vi "EnergyMeter Read.vi"(3 "错误输入（无错误）":errorcluster) -> (0 "通信正常？":bool, 1 "错误输出":errorcluster, 2 "能量计读数":string)   [LabVIEW 2018]
uses:
  InOut/Reslut.vi
panel:
  out "Unit":string
  out "能量计输出":dbl
  out "结果字符串":string
  out "数据输出":string
  # "通道A为功率计"
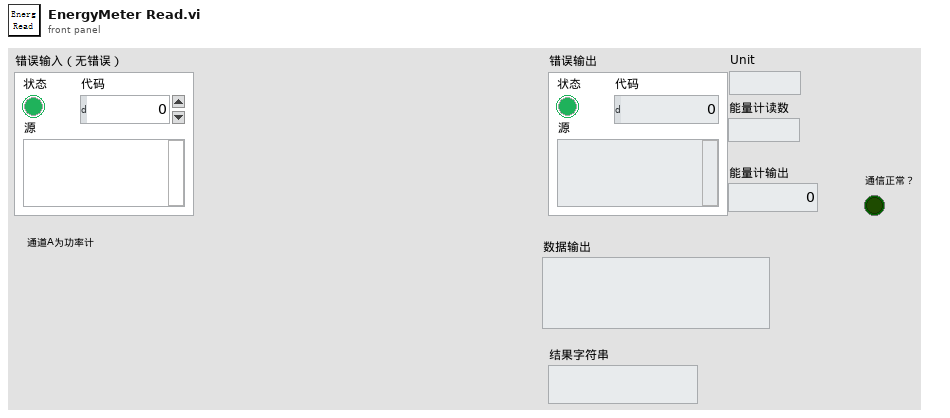
[diagram p1: front panel]
types:
  T1 = enum16{"Standard", "Buffered", "CRLF", "Immediate"}
  T2 = typedef "IMAQ Image.ctl" = refnum<image>
  T3 = cluster{"示波器":cluster{"Channel (0:Channel 1)":enum16{"Channel 1", "Channel 2", "Channel 3", "Channel 4"}, "电压范围":dbl, "触发电压":dbl, "时间范围":dbl, " 示波器VISA":refnum<visa-resource-name>}, "光谱仪":cluster{"Channel (0:Channel 1)":enum16{"Channel 1", "Channel 2", "Channel 3", "Channel 4"}, "电压范围":u64, "触发电压":u64, "时间范围":u64}, " 近场相机":cluster{"曝光时间":i32, "模拟增益":i32, "控制套接字":i32, "IP 地址":string, " 采集套接字":i32, "  版本号":i32, "ImageData":T2, "  增益最大":i32, "  增益最小":i32, " 曝光最大":i32, " 曝光最小":i32, " 帧速":i32, " 同步切换":i32, "  曝光缩放":i32}, " 偏振仪":cluster{"电压范围":u64, "触发电压":u64, "时间范围":u64, "波长范围":enum16{"可见光 400-700nm", "近红外 700-1100nm"}}, " 功率计":cluster{"通道":enum16{"Channel 1", "Channel 2"}, "工作波长":u32, "单位":u64, "时间范围":u64, "IP地址":string, "端口":u32}, "能量计":cluster{"通道":enum16{"Channel 1", "Channel 2"}, "工作波长":u32, "单位":u64, "时间范围":u64, "IP地址":string, "端口":u32, "能量计量程":enum16{"200uJ", "20uJ", "2uJ", "200nJ"}}, "电机":cluster{"Channel (0:Channel 1)":enum16{"Channel 1", "Channel 2", "Channel 3", "Channel 4"}, "电压范围":u64, "触发电压":u64, "时间范围":u64}, " 远场相机":cluster{"曝光时间":i32, "模拟增益":i32, "控制套接字":i32, "IP 地址":string, " 采集套接字":i32, "  版本号":i32, "ImageData":T2, "  增益最大":i32, "  增益最小":i32, " 曝光最大":i32, " 曝光最小":i32, " 帧速":i32, " 同步切换":i32, "  曝光缩放":i32}}
  T4 = cluster{"能量计结果":string, "功率计结果":string, "能量计单位":string, " 功率计单位":string}
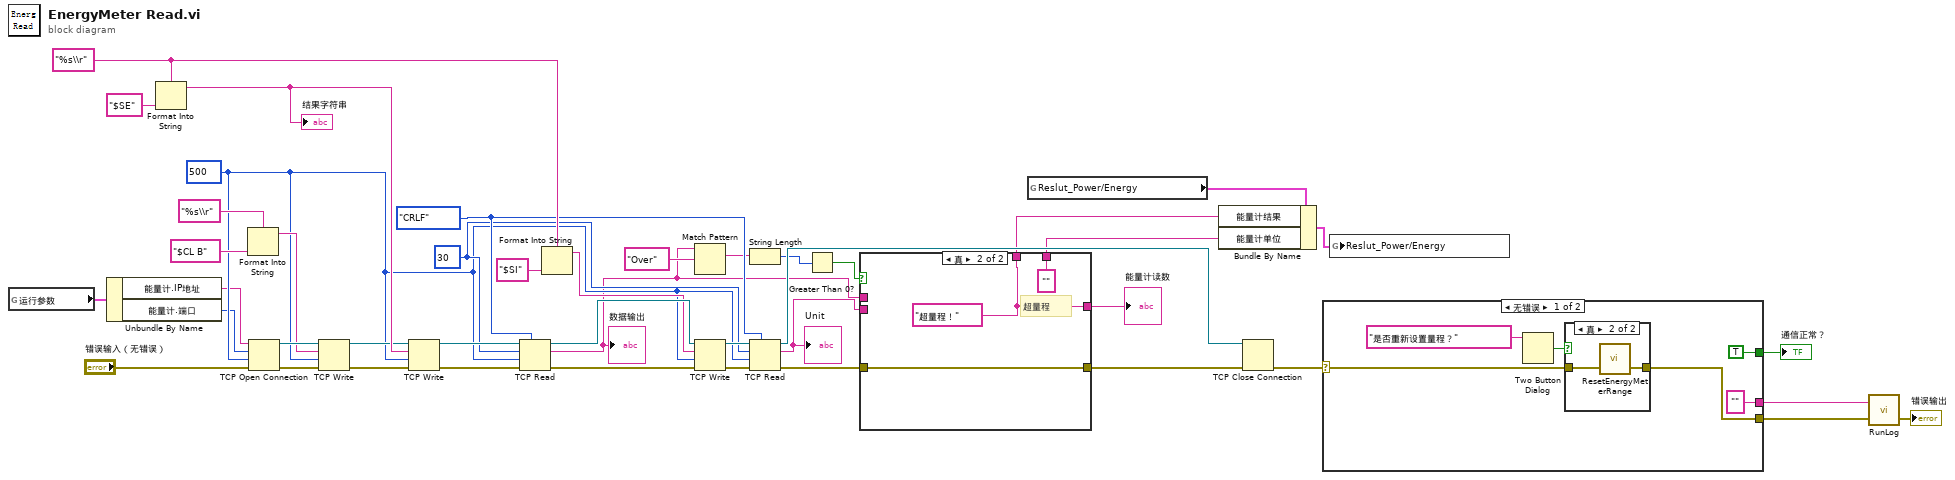
[diagram p0: block diagram]
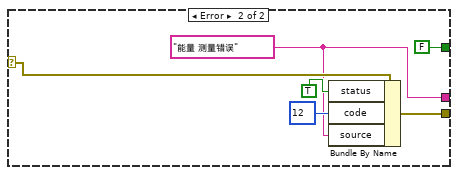
[diagram p3: hidden frame]
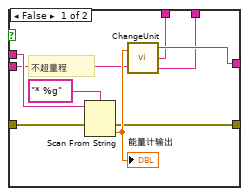
[diagram p4: hidden frame]
diagram:
  w23 = 30 ("读取的字节")
  w22 = 500 ("超时毫秒(25000)")
  w26 = T1."CRLF" ("模式（标准）")
  w29 = "%s\\r" ("格式字符串")
  n1 = global read "参数.vi" "运行参数"() -> (w20:T3)
  n2 = Unbundle By Name(w20) -> ("能量计.IP地址"=w19:string, "能量计.端口"=w18:u32)
  n3 = Format Into String(format string=w29, "$SE" ("输入 1")) -> (resulting string=w43:string)  [unwired: 2 in, 1 out]
  "结果字符串" <- w43
  n4 = Format Into String(format string="%s\\r" ("格式字符串"), "$CL B" ("输入 1")) -> (resulting string=w37:string)  [unwired: 2 in, 1 out]
  n5 = TCP Open Connection(address=w19, remote port or service name=w18, timeout ms (60000)=w22, error in (no error)="错误输入（无错误）") -> (connection ID=w38:refnum<k5>, error out=w36:errorcluster)  [unwired: 1 in]
  n6 = TCP Write(connection ID=w38, data in=w37, error in (no error)=w36, 9:w22) -> (connection ID out=w35:refnum<k5>, error out=w34:errorcluster)  [unwired: 1 out]
  n7 = TCP Write(connection ID=w35, data in=w43, error in (no error)=w34, 9:w22) -> (connection ID out=w42:refnum<k5>, error out=w41:errorcluster)  [unwired: 1 out]
  n8 = TCP Read(connection ID=w42, bytes to read=w23, error in (no error)=w41, 7:w26, 9:w22) -> (connection ID out=w31:refnum<k5>, data out=w13:string, error out=w30:errorcluster)
  "数据输出" <- w13
  n9 = Format Into String(format string=w29, "$SI" ("输入 1")) -> (resulting string=w27:string)  [unwired: 2 in, 1 out]
  n10 = Match Pattern(string=w13, regular expression="Over" ("正则表达式")) -> (match substring=w16:string)  [unwired: 1 in, 3 out]
  n11 = TCP Write(connection ID=w31, data in=w27, error in (no error)=w30, 9:w22) -> (connection ID out=w25:refnum<k5>, error out=w24:errorcluster)  [unwired: 1 out]
  n12 = String Length(string=w16) -> (length=w15:i32)
  n13 = TCP Read(connection ID=w25, bytes to read=w23, error in (no error)=w24, 7:w26, 9:w22) -> (connection ID out=w21:refnum<k5>, data out=w12:string, error out=w11:errorcluster)
  "Unit" <- w12
  n14 = Greater Than 0?(x=w15) -> (x > 0?=w14:bool)
  n15 = case shown="真" w14 {
    tunnel: w13 -> [w52 _]
    tunnel: [w50 w55] -> w9
    tunnel: w12 -> [w49 _]
    tunnel: w11 -> [w48 w56]
    tunnel: [w47 w56] -> w10
    tunnel: [w46 w55] -> w3
    tunnel: [w45 "" ("UintOut")] -> w2
    frame False {
      # "不超量程"
      n16 = Scan From String(format string="* %g" ("格式字符串"), input string=w52, error in=w48) -> (error out=w47:errorcluster, output 1=w51:dbl)  [unwired: 2 in, 2 out]
      "能量计输出" <- w51
      n17 = call "ChangeUnit.vi"("change in"=w51, "unit in"=w49) -> ("change out"=w50:string, "DataOut"=w46:string, "UintOut"=w45:string)
    }
    frame True {
      w55 = "超量程！" ("正则表达式")
      # "超量程"
    }
  }
  "能量计读数" <- w9
  n18 = global read "Reslut.vi" "Reslut_Power/Energy"() -> (w4:T4)
  n19 = Bundle By Name(cluster=w4, "能量计结果"=w3, "能量计单位"=w2) -> (w1:T4)
  n20 = TCP Close Connection(connection ID=w21, error in (no error)=w10) -> (error out=w32:errorcluster)  [unwired: 1 in, 1 out]
  n21 = case shown="无错误" w32 {
    selector: w32 -> [w58 w70]
    tunnel: [TRUE FALSE] -> w8
    tunnel: [w57 w66] -> w7
    tunnel: ["" ("source") w67] -> w6
    frame No Error {
      n22 = Two Button Dialog(message="是否重新设置量程？" ("消息")) -> (T button?=w60:bool)  [unwired: 2 in]
      n23 = case shown="真" w60 {
        tunnel: w58 -> [w63 w65]
        tunnel: [w63 w64] -> w57
        frame False {
        }
        frame True {
          n24 = call "ResetEnergyMeterRange.vi"("错误输入（无错误）"=w65) -> ("错误输出"=w64:errorcluster)  [unwired: 2 in]
        }
      }
    }
    frame Error {
      w67 = "能量 测量错误" ("source")
      n25 = Bundle By Name(cluster=w70, "status"=TRUE, "code"=12, "source"=w67) -> (w66:errorcluster)
    }
  }
  "通信正常？" <- w8
  n26 = global write "Reslut.vi" "Reslut_Power/Energy"(w1) -> ()
  n27 = call "RunLog.vi"("error in"=w7, "Message"=w6) -> ("error out"=→"错误输出":errorcluster)  [unwired: 1 in]
